vi "Process Gas Select Command (SubVI).vi"(4 "Gas Select In":string, 6 "Address":string, 8 "error in (no error)":errorcluster, 11 "VISA Refnum in":refnum<visa-resource-name>) -> (0 "error out":errorcluster, 2 "Gas Select Out":string, 3 "VISA Refnum out":refnum<visa-resource-name>)   [LabVIEW 2020]
doc: "Reads currently selected Gas name from the instrument (if \"Gas Select In\" terminal is not wired). Writes specified Gas number to the instrument (\"Gas Select In\" terminal need to be wired with desired gas index decimal string)."
uses:
  <vilib>/Instr/_visa.llb/VISA Flush IO Buffer Mask.ctl
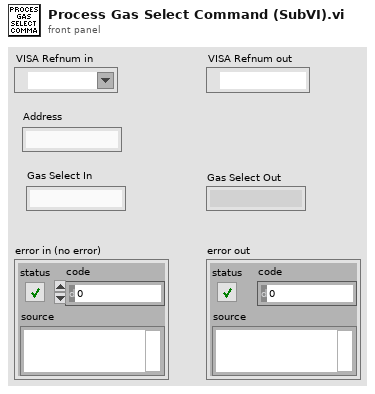
[diagram p1: front panel]
types:
  T1 = typedef "VISA Flush IO Buffer Mask.ctl" = u16
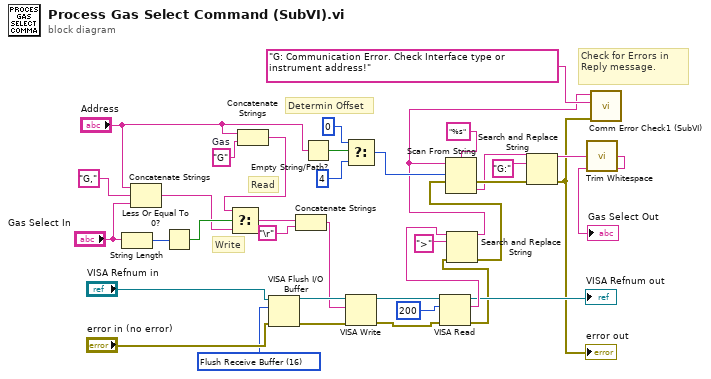
[diagram p0: block diagram]
diagram:
  w25 = "G"  # Gas
  w26 = T1 16 items=["Flush Receive Buffer"=16, "Write Transmit Buffer to Device"=32, "Flush Receive Buffer (No I/O)"=64, "Flush Transmit Buffer"=128] ("Mask")
  # "Write"
  # "Read"
  # "Check for Errors in Reply message."
  # "Determin Offset"
  n1 = String Length(string="Gas Select In") -> (length=w6:i32)
  n2 = Concatenate Strings("Address", "G,", "Gas Select In") -> (w2:string)
  n3 = Less Or Equal To 0?(x=w6) -> (x <= 0?=w5:bool)
  n4 = Concatenate Strings("Address", w25) -> (w10:string)
  n5 = Select(t=w10, s=w5, f=w2) -> (s? t:f=w9:string)
  n6 = VISA Flush I/O Buffer(VISA resource name="VISA Refnum in", mask (16)=w26, error in (no error)="error in (no error)") -> (VISA resource name out=w31:refnum<visa-resource-name>, error out=w8:errorcluster)
  n7 = Concatenate Strings(w9, "\r") -> (w30:string)
  n8 = Empty String/Path?(string/path="Address") -> (empty?=w22:bool)
  n9 = Select(t=0, s=w22, f=4) -> (s? t:f=w15:i32)
  n10 = VISA Write(VISA resource name=w31, write buffer=w30, error in (no error)=w8) -> (VISA resource name out=w33:refnum<visa-resource-name>, error out=w37:errorcluster)  [unwired: 1 out]
  n11 = VISA Read(VISA resource name=w33, byte count=200, error in (no error)=w37) -> (VISA resource name out=→"VISA Refnum out":refnum<visa-resource-name>, read buffer=w36:string, error out=w18:errorcluster)  [unwired: 1 out]
  n12 = Search and Replace String(input string=w36, search string=">", error in=w18) -> (result string=w12:string, error out=w17:errorcluster)  [unwired: 5 in, 2 out]
  n13 = Scan From String(format string="%s", input string=w12, initial scan location=w15, error in=w17) -> (error out=w16:errorcluster, output 1=w14:string)  [unwired: 1 in, 2 out]
  n14 = Search and Replace String(input string=w14, search string="G:", error in=w16) -> (result string=w23:string, error out=w11:errorcluster)  [unwired: 5 in, 2 out]
  "error out" <- w11
  n15 = call <vilib>:"Trim Whitespace.vi"("string"=w23) -> ("trimmed string"=→"Gas Select Out":string)  [unwired: 1 in]
  n16 = call "Comm Error Check1 (SubVI).vi"("error in (no error)"=w11, "Error Source String"="G: Communication Error. Check Interface type or instrument address!", "result string"=w12) -> ()  [unwired: 9 in]
